vi "ex4.vi"() -> ()   [LabVIEW 2022 SP3]
uses:
  #typedef_ex4.ctl
  #typdef_ex4_states.ctl
panel:
  out "Info":T1
  in  "Stop":bool
  in  "Run Cleaning":bool
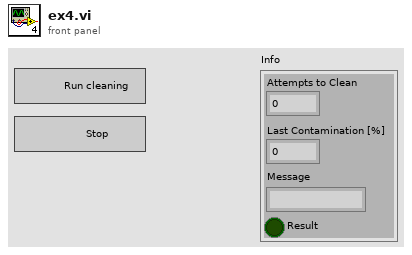
[diagram p1: front panel]
types:
  T1 = typedef "#typedef_ex4.ctl" = cluster{"Attempts to Clean":dbl, "Last Contamination [%]":dbl, "Message":string, "Result":bool}
  T2 = typedef "#typdef_ex4_states.ctl" = enum16{"Reset Values", "Exit", "Initialization", "Idle", "Contamination Check", "Refresh GUI", "Cleaning Water", "Error Handler", "Too Much Tries"}
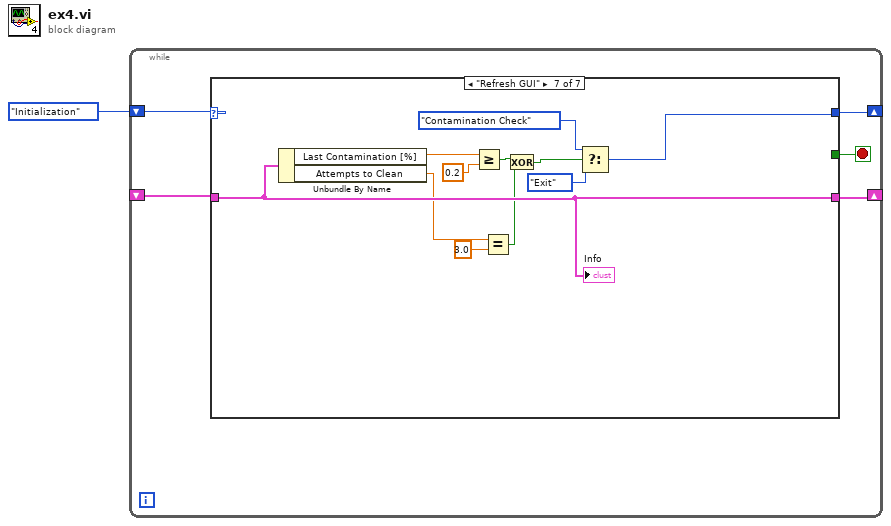
[diagram p0: block diagram]
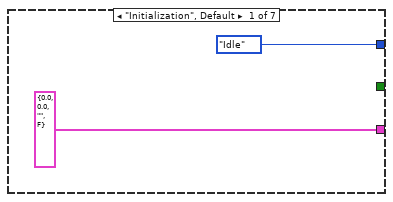
[diagram p2: hidden frame]
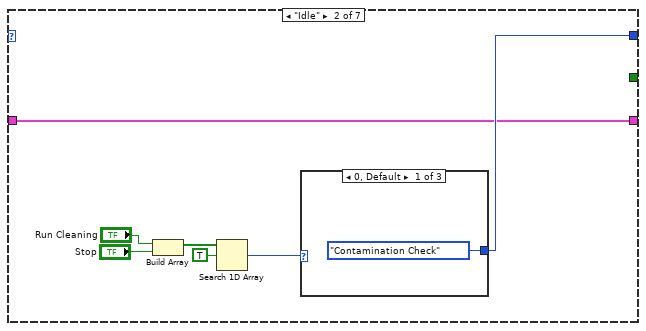
[diagram p3: hidden frame]
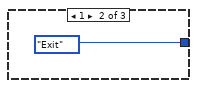
[diagram p4: hidden frame]
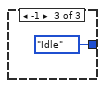
[diagram p5: hidden frame]
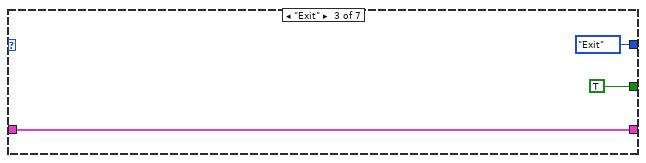
[diagram p6: hidden frame]
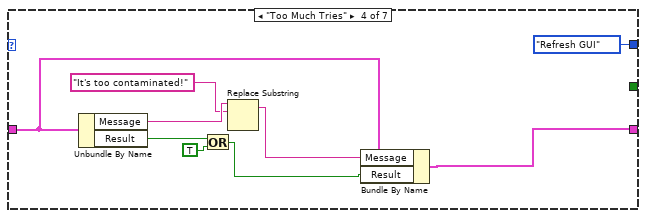
[diagram p7: hidden frame]
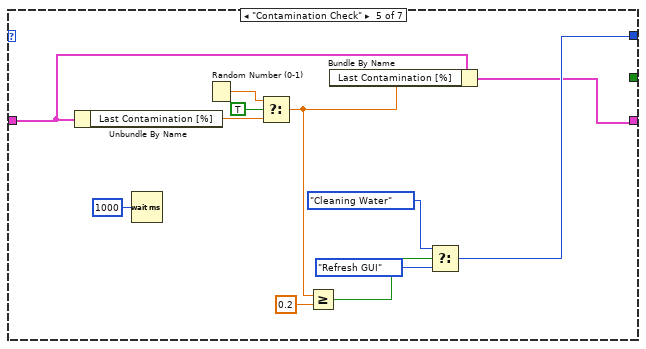
[diagram p8: hidden frame]
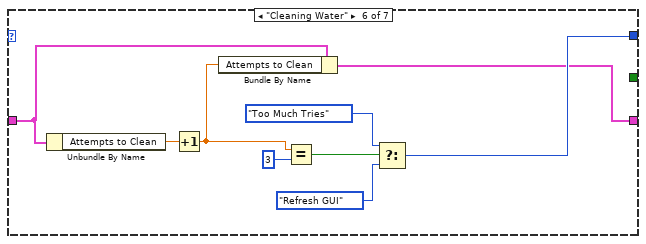
[diagram p9: hidden frame]
diagram:
  n1 = while {
    shift-right: [w5] -> _
    shift-left: #typdef_ex4_states."Initialization" ("Enum") -> [w6]
    shift-right: [w3] -> _
    shift-left: _ -> [w4]
    stop <- w2 stop-if-true
    n2 = case shown="\"Refresh GUI\"" w6 {
      tunnel: [#typdef_ex4_states."Idle" ("Enum") w10 #typdef_ex4_states."Exit" ("Enum") #typdef_ex4_states."Refresh GUI" ("Enum") w33 w47 w57] -> w5
      tunnel: w4 -> [_ w9 w20 w27 w36 w44 w62]
      tunnel: [T1 {"Attempts to Clean"=0.0, "Last Contamination [%]"=0.0, "Message"="", "Result"=FALSE} ("Cluster") w9 w20 w25 w32 w43 w62] -> w3
      tunnel: [_ _ TRUE _ _ _ _] -> w2
      frame "Initialization", Default {
      }
      frame "Idle" {
        n3 = Build Array("Run Cleaning", "Stop") -> (w13:bool[])
        n4 = Search 1D Array(1D array=w13, element=TRUE) -> (index of element=w11:i32)  [unwired: 1 in]
        n5 = case shown="0, Default" w11 {
          tunnel: [#typdef_ex4_states."Contamination Check" ("Enum") #typdef_ex4_states."Exit" ("Enum") #typdef_ex4_states."Idle" ("Enum")] -> w10
          frame 0, Default {
          }
          frame 1 {
          }
          frame -1 {
          }
        }
      }
      frame "Exit" {
      }
      frame "Too Much Tries" {
        n6 = Unbundle By Name(w27) -> ("Message"=w24:string, "Result"=w29:bool)
        n7 = Or(x=w29, y=TRUE) -> (x .or. y?=w26:bool)
        n8 = Replace Substring(4:"It's too contaminated!" ("substring (\"\")"), 5:w24) -> (1:w22:string)  [unwired: 2 in, 1 out]
        n9 = Bundle By Name(cluster=w27, "Message"=w22, "Result"=w26) -> (w25:T1)
      }
      frame "Contamination Check" {
        n10 = Unbundle By Name(w36) -> ("Last Contamination [%]"=w39:dbl)
        n11 = Wait (ms)(milliseconds to wait=u32 1000) -> ()  [unwired: 1 out]
        n12 = Random Number (0-1)() -> (number: 0 to 1=w37:dbl)
        n13 = Select(t=w37, s=TRUE, f=w39) -> (s? t:f=w34:dbl)
        n14 = Greater Or Equal?(x=w34, y=0.2) -> (x >= y?=w40:bool)
        n15 = Bundle By Name(cluster=w36, "Last Contamination [%]"=w34) -> (w32:T1)
        n16 = Select(t=#typdef_ex4_states."Cleaning Water" ("Enum"), s=w40, f=#typdef_ex4_states."Refresh GUI" ("Enum")) -> (s? t:f=w33:T2)
      }
      frame "Cleaning Water" {
        n17 = Unbundle By Name(w44) -> ("Attempts to Clean"=w46:dbl)
        n18 = Increment(x=w46) -> (x+1=w45:dbl)
        n19 = Bundle By Name(cluster=w44, "Attempts to Clean"=w45) -> (w43:T1)
        n20 = Equal?(x=w45, y=3) -> (x = y?=w50:bool)
        n21 = Select(t=#typdef_ex4_states."Too Much Tries" ("Enum"), s=w50, f=#typdef_ex4_states."Refresh GUI" ("Enum")) -> (s? t:f=w47:T2)
      }
      frame "Refresh GUI" {
        n22 = Unbundle By Name(w62) -> ("Last Contamination [%]"=w61:dbl, "Attempts to Clean"=w56:dbl)
        n23 = Greater Or Equal?(x=w61, y=0.2) -> (x >= y?=w54:bool)
        n24 = Equal?(x=w56, y=3.0) -> (x = y?=w53:bool)
        n25 = Exclusive Or(1:w53, 2:w54) -> (0:w52:bool)
        n26 = Select(t=#typdef_ex4_states."Contamination Check" ("Enum"), s=w52, f=#typdef_ex4_states."Exit" ("Enum")) -> (s? t:f=w57:T2)
        "Info" <- w62
      }
    }
  }
